vi "Tool Connect.vi"(8 "error in (no error)":errorcluster, 10 "Tool Operation Config":T1={"Use Tool Cfg"=FALSE, "Use Tool Cal"=FALSE, "Fake Data?"=FALSE, "Mode"=-2, "Array Subset Length"=30, "nArrays to Read"=2, "Full Array Read Length"=500, "nSubarrays/Sensor"=0}) -> (0 "error out":errorcluster, 1 "Connected":bool, 2 "Tool Operation Config out":T1={"Use Tool Cfg"=FALSE, "Use Tool Cal"=FALSE, "Fake Data?"=FALSE, "Mode"=-2, "Array Subset Length"=30, "nArrays to Read"=2, "Full Array Read Length"=500, "nSubarrays/Sensor"=0}, 4 "No Cfg Data?":bool, 5 "Tool Serial Number":u16, 7 "Tool Type":u16)   [LabVIEW 2015, in "Tool Module.lvlib"]
uses:
  Tool Module.lvlib
  Tool Config/_Tool Operation Config Cluster--typedef.ctl
  Tool Typedefs/_Data Stream Fmt Params Cluster--typedef.ctl
  ToolModGLOB.vi
  Tool Interface/Tool Interface.lvlib
  Tool Config/Tool Cfg.lvlib
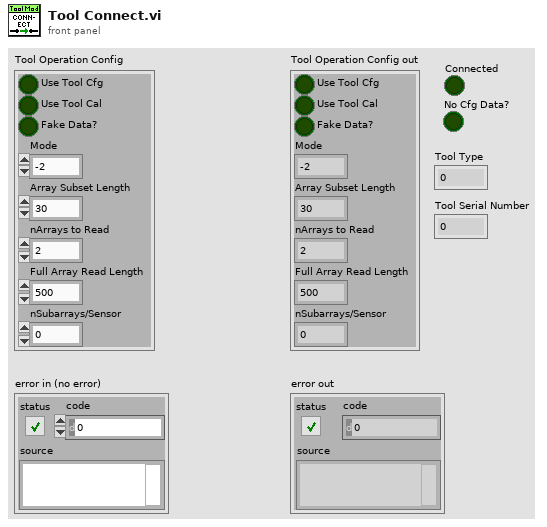
[diagram p1: front panel]
types:
  T1 = typedef "Tool Cfg.lvlib/_Tool Operation Config Cluster--typedef.ctl" = cluster{"Use Tool Cfg":bool, "Use Tool Cal":bool, "Fake Data?":bool, "Mode":i16, "Array Subset Length":i16, "nArrays to Read":i16, "Full Array Read Length":i16, "nSubarrays/Sensor":i16}
  T2 = typedef "_Data Stream Fmt Params Cluster--typedef.ctl" = cluster{"Samples per Block":i32, "Raw Data Status Len":i32, "Fltr Data Status Len":i32}
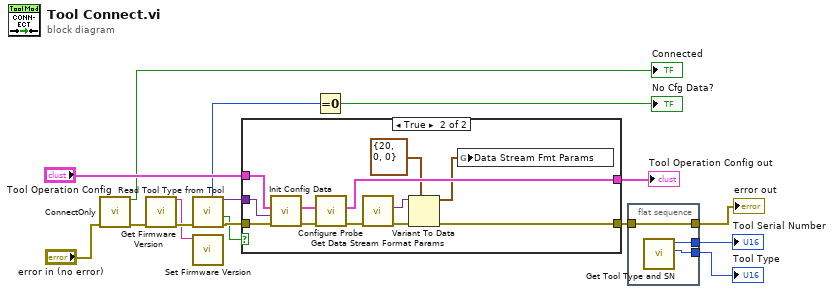
[diagram p0: block diagram]
diagram:
  n1 = call "ConnectOnly.vi"("error in (no error)"="error in (no error)") -> ("error out"=w9:errorcluster, "Success"=→"Connected":bool)  [unwired: 9 in]
  n2 = call "Get Firmware Version.vi"("error in (no error)"=w9) -> ("error out"=w8:errorcluster, "Firmware Version String"=w2:string)  [unwired: 9 in]
  n3 = call "Read Tool Type from Tool.vi"("error in (no error)"=w8) -> ("error out"=w6:errorcluster, "Success"=w5:bool, "Message Data"=w3:variant, "Data Count"=w4:i32)  [unwired: 6 in, 1 out]
  n4 = call "Set Firmware Version.vi"("Firmware Version String"=w2) -> ()  [unwired: 11 in]
  n5 = case shown="True" w5 {
    tunnel: w6 -> [w18 w30]
    tunnel: "Tool Operation Config" -> [w17 w29]
    tunnel: [w18 w22] -> w11
    tunnel: [w17 w28] -> w15
    tunnel: w3 -> [_ w25]
    frame False {
    }
    frame True {
      n6 = call "Init Config Data.vi"("error in (no error)"=w30, "Config Data in"=w25, "Tool Operation Config"=w29) -> ("error out"=w26:errorcluster, "Tool Op Cfg out"=w27:T1)  [unwired: 7 in]
      n7 = call "Configure Probe.vi"("error in (no error)"=w26, "Tool Operation Config"=w27) -> ("error out"=w24:errorcluster, "Tool Operation Config out"=w28:T1)  [unwired: 8 in]
      n8 = call "Get Data Stream Format Params.vi"("error in (no error)"=w24) -> ("error out"=w23:errorcluster, "Message Data"=w21:variant)  [unwired: 7 in, 2 out]
      n9 = Variant To Data(error in=w23, type=T2 {"Samples per Block"=20, "Raw Data Status Len"=0, "Fltr Data Status Len"=0} ("_Acq  Process Params Cluster--typedef"), Variant=w21) -> (data=w19:T2, error out=w22:errorcluster)
      n10 = global write "ToolModGLOB.vi" "Data Stream Fmt Params"(w19) -> ()
    }
  }
  "Tool Operation Config out" <- w15
  n11 = Equal To 0?(x=w4) -> (x = 0?=→"No Cfg Data?":bool)
  n12 = flat-sequence {
    tunnel: w11 -> [w33]
    tunnel: [w33] -> w10
    tunnel: [w32] -> w13
    tunnel: [w31] -> w12
    frame #0 {
      n13 = call "Get Tool Type and SN.vi"() -> ("Tool SN"=w31:u16, "Tool Type"=w32:u16)  [unwired: 10 in]
    }
  }
  "error out" <- w10
  "Tool Type" <- w12
  "Tool Serial Number" <- w13
